vi "editDialogDontUse.vi"(0 "reference":refnum<class "CallNode.lvclass">, 1 "insidePackageNode":bool, 5 "error in (no error)":errorcluster) -> (14 "reference out":refnum<class "CallNode.lvclass">, 15 "changeConnection":T1, 16 "cancel":bool, 19 "error out":errorcluster)   [LabVIEW 2014, in "CallNode.lvclass"]
doc: "Edit Dialog"
uses:
  <resource>/Framework/Providers/Open_GDS/UML/CallNode_class/CallNode.lvclass
  <resource>/Framework/Providers/Open_GDS/UML/AbstractNode_class/private/NodeConnectionStatsType.ctl
  <resource>/Framework/Providers/Open_GDS/UML/AbstractNode_class/AbstractNode.lvclass
panel:
  in  "Cancel Button":bool
  in  "OK Button":bool
  in  "Open bottom":bool
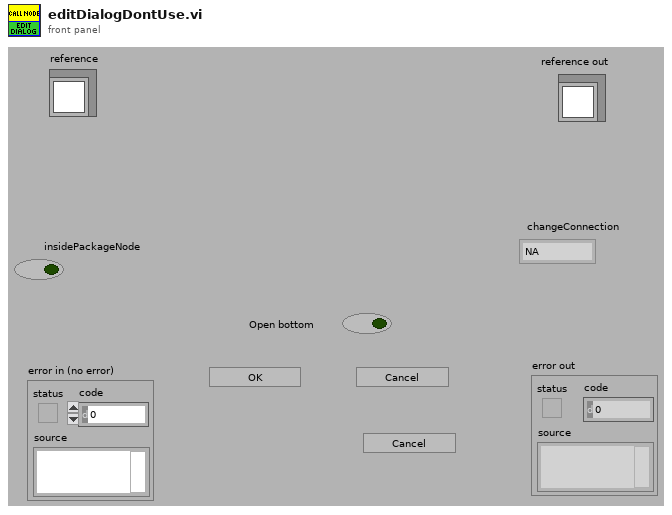
[diagram p1: front panel]
types:
  T1 = typedef "AbstractNode.lvclass/NodeConnectionStatsType.ctl" = enum16{"NA", "Connect", "DisConnect"}
  T2 = typedef "CallNode.lvclass/ObjectAttributes.ctl" = cluster{"objectCallNodeRef":refnum<class "AbstractNode.lvclass">, "signaled":bool, "openBottom":bool, "DEFAULT_WIDTH":i32, "DEFAULT_HEIGHT":i32, "CALL_YGAP":i32}
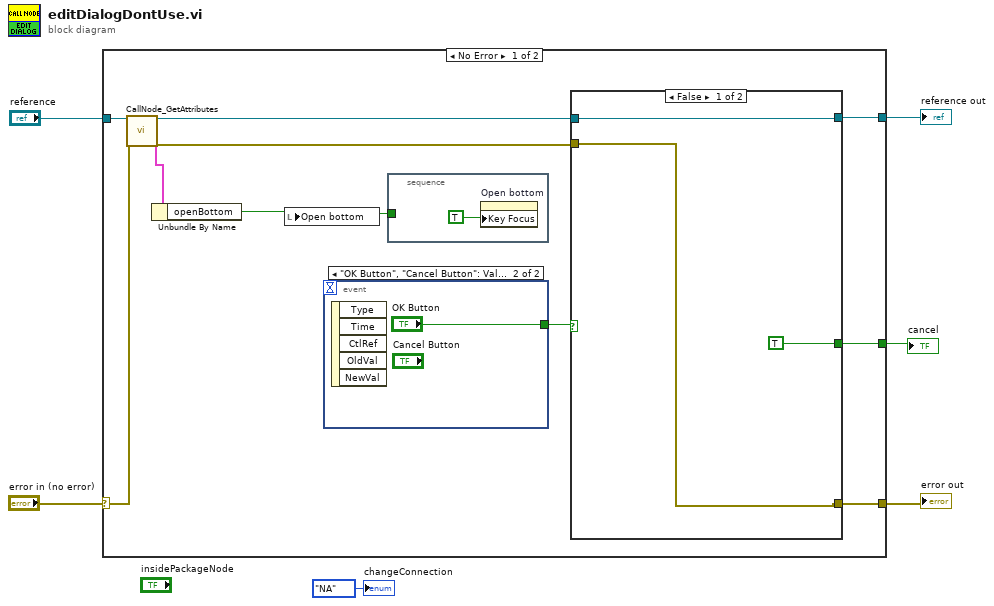
[diagram p0: block diagram]
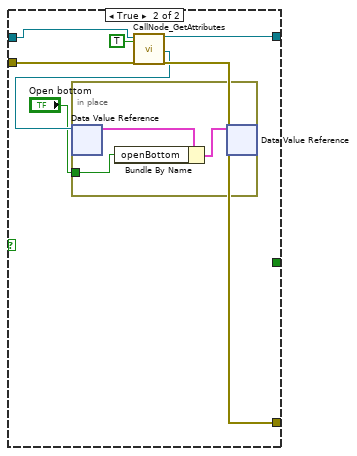
[diagram p2: hidden frame]
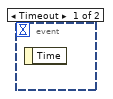
[diagram p3: hidden frame]
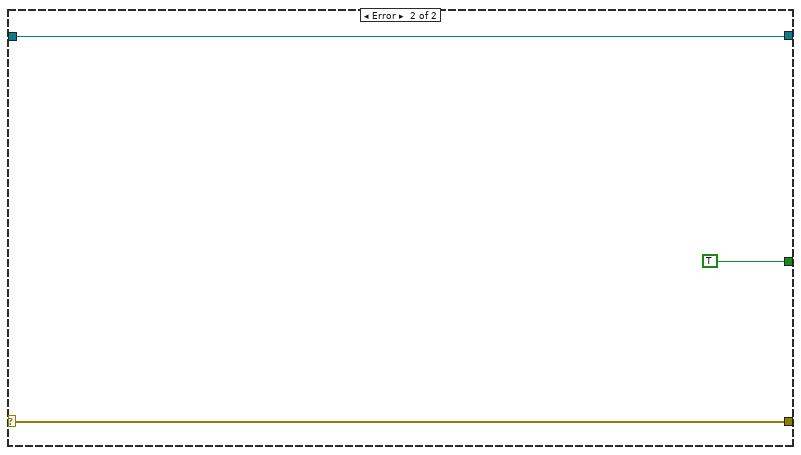
[diagram p4: hidden frame]
diagram:
  n1 = case shown="No Error" "error in (no error)" {
    selector: "error in (no error)" -> [w12 w33]
    tunnel: "reference" -> [w13 w34]
    tunnel: [w16 w33] -> w4
    tunnel: [w15 w34] -> w3
    tunnel: [w10 TRUE ("Key Focus")] -> w1
    frame No Error {
      n2 = call <resource>:"CallNode_GetAttributes.vi"("reference in"=w13, "error in (no error)"=w12) -> ("reference out"=w14:refnum<class "CallNode.lvclass">, "Data"=w7:T2, "error out"=w8:errorcluster)  [unwired: 1 in, 14 out]
      n3 = Unbundle By Name(w7) -> ("openBottom"=w9:bool)
      n4 = local write "Open bottom"(w9) -> ()
      n5 = event shown="[1] \"OK Button\", \"Cancel Button\": Value Change" {
        selector: _ -> [_ _]
        dyn-events: _ -> [_ _]
        timeout: _ -> [_ _]
        tunnel: [_ "OK Button"] -> w11
        event Timeout {
          n6 = event-data() -> ()  [unwired: 2 out]
        }
        event "OK Button", "Cancel Button": Value Change {
          n7 = event-data() -> ()  [unwired: 6 out]
        }
      }
      n8 = stacked-sequence {
        tunnel: w9 -> [_]
        frame #0 {
          n9 = property on="Open bottom" class="Bool (strict)"("Key Focus"=TRUE) -> ()  [unwired: 2 in, 2 out]
        }
      }
      n10 = case shown="False" w11 {
        tunnel: [w17 w26] -> w16
        tunnel: [w19 w25] -> w15
        tunnel: w14 -> [w19 w24]
        tunnel: [TRUE ("Key Focus") _] -> w10
        tunnel: w8 -> [w17 w23]
        frame False {
        }
        frame True {
          n11 = call <resource>:"CallNode_GetAttributes.vi"("reference in"=w24, "OnlyGetDvrReference(False)"=TRUE, "error in (no error)"=w23) -> ("reference out"=w25:refnum<class "CallNode.lvclass">, "DataRef"=w21:refnum<data-value>, "error out"=w26:errorcluster)  [unwired: 13 in, 1 out]
          n12 = in-place {
            in-place-border: "Open bottom" -> [w28]
            n13 = in-place-dvr #1(w21) -> (w29:T2)  [unwired: 1 out]
            n14 = Bundle By Name(cluster=w29, "openBottom"=w28) -> (w27:T2)
            n15 = in-place-dvr #1(w27) -> ()  [unwired: 2 out]
          }
        }
      }
    }
    frame Error {
    }
  }
  "reference out" <- w3
  "error out" <- w4
  "cancel" <- w1
  "changeConnection" <- NodeConnectionStatsType."NA" ("changeConnection")
